vi "create_full_request_data.vi"(0 "llm_openai_chatmodels in":refnum<class "llm_gemini_chatmodels.lvclass">, 5 "Messages":refnum<class "abstract_message_base.lvclass">[](array[class]), 11 "error in (no error)":errorcluster) -> (4 "llm_openai_chatmodels out":refnum<class "llm_gemini_chatmodels.lvclass">, 6 "Request Data":string, 15 "error out":errorcluster)   [LabVIEW 2020, in "llm_gemini_chatmodels.lvclass"]
uses:
  llm_gemini_chatmodels.lvclass
  C:/Users/venkatesh.chandragir/Downloads/labview-llm-libraries-users-nigharikkha-vlm_support/src/models/abstract_llm_base/abstract_llm_base.lvclass
  abstract_message_base/abstract_message_base.lvclass
  utils/gemini_chatmodel_request_data.ctl
  message_text/message_text.lvclass
  message_image/message_image.lvclass
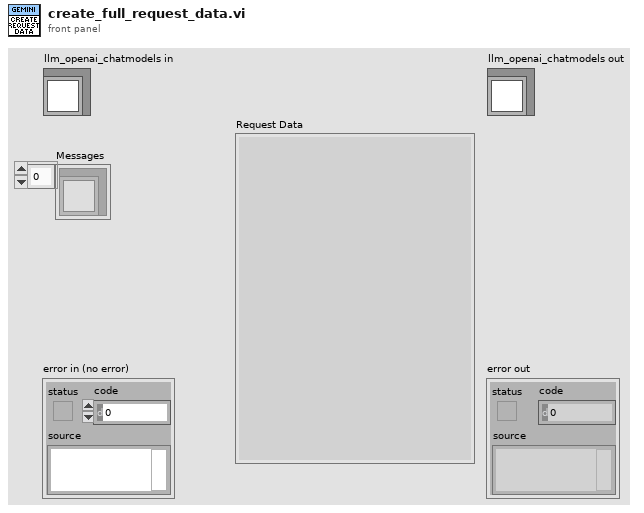
[diagram p1: front panel]
types:
  T1 = cluster{"role":string, "parts":cluster{"text":string}[]}[]
  T2 = typedef "llm_gemini_chatmodels.lvclass/gemini_chatmodel_request_data.ctl" = cluster{"contents":cluster{"role":string, "parts":cluster{"text":string}[]}[], "generation_config":cluster{"temperature":dbl, "maxOutputTokens":u32, "topP":dbl}}
  T3 = typedef "message_text.lvclass/message.ctl" = cluster{"role":string, "content":string[]}
  T4 = typedef "message_image.lvclass/message.ctl" = cluster{"role":string, "content_text":string[], "content_images":path[]}
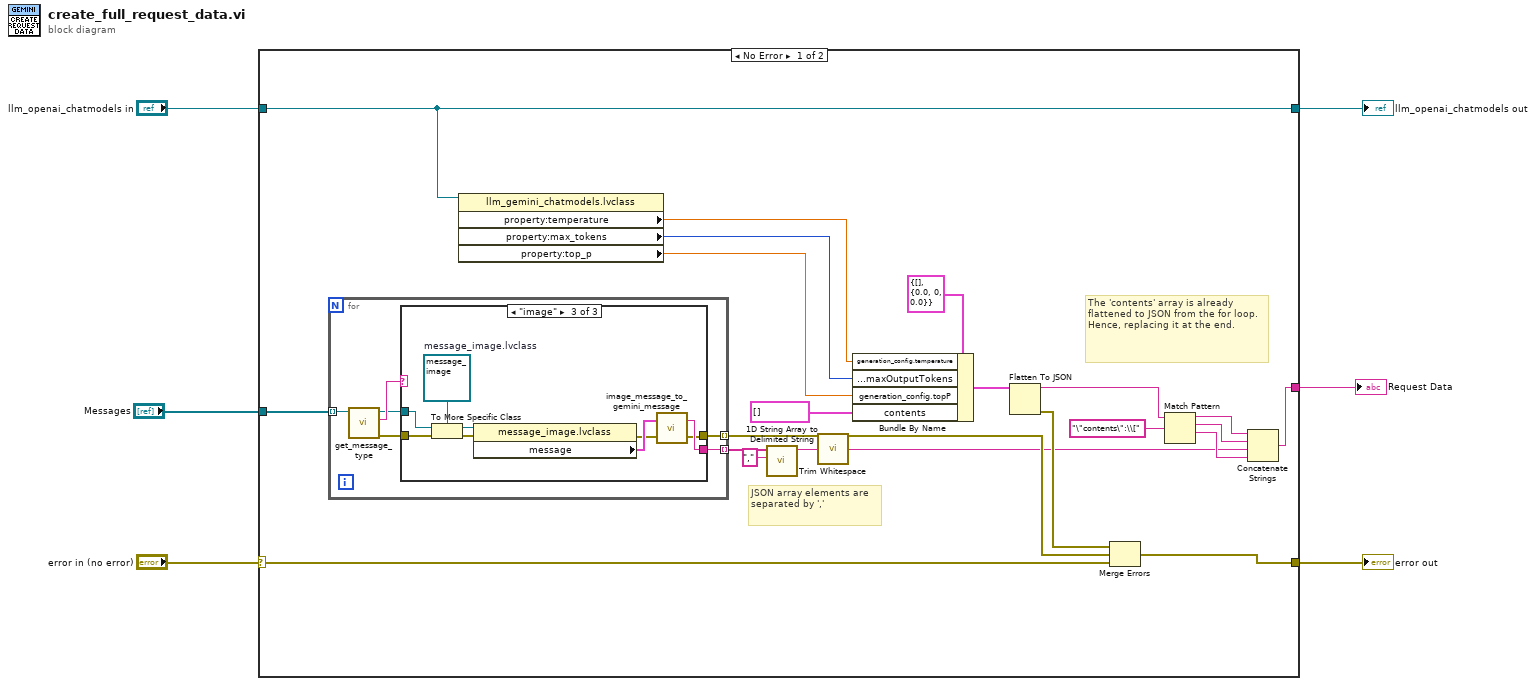
[diagram p0: block diagram]
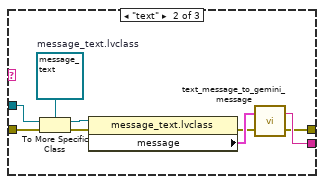
[diagram p3: hidden frame]
diagram:
  n1 = case shown="No Error" "error in (no error)" {
    selector: "error in (no error)" -> [w28 w55]
    tunnel: [w25 w55] -> w5
    tunnel: [w22 w54] -> w3
    tunnel: "llm_openai_chatmodels in" -> [w22 w54]
    tunnel: "Messages" -> [w27 _]
    tunnel: [w11 _] -> w1
    frame No Error {
      # "JSON array elements are separated by ','"
      # "The 'contents' array is already flattened to JSON from the for loop.\nHence, replacing it at the end."
      n2 = for {
        tunnel: w27 -> [w34] mode=indexing
        tunnel: [w30] -> w24 mode=indexing
        tunnel: [w29] -> w8 mode=indexing
        n3 = call-dynamic "get_message_type.vi"("abstract_message_base in"=w34) -> ("error out"=w31:errorcluster, "Type"=w33:string, "abstract_message_base out"=w32:refnum<class "abstract_message_base.lvclass">)  [unwired: 8 in]
        n4 = case shown="\"image\"" w33 {
          tunnel: w32 -> [_ w43 w52]
          tunnel: w31 -> [w35 w44 w53]
          tunnel: [w35 w36 w45] -> w30
          tunnel: [_ w38 w47] -> w29
          frame Default {
          }
          frame "text" {
            w42 = refnum<class "message_text.lvclass"> refnum  # message_text.lvclass
            n5 = To More Specific Class(target class=w42, reference=w43, error in=w44) -> (specific class reference=w41:refnum<class "message_text.lvclass">, error out=w40:errorcluster)
            n6 = property class="message_text.lvclass"(reference=w41, error in=w40) -> (error out=w37:errorcluster, "message"=w39:T3)  [unwired: 1 out]
            n7 = call "text_message_to_gemini_message.vi"("error in (no error)"=w37, "message"=w39) -> ("error out"=w36:errorcluster, "Content (JSON)"=w38:string)
          }
          frame "image" {
            w49 = refnum<class "message_image.lvclass"> refnum  # message_image.lvclass
            n8 = To More Specific Class(target class=w49, reference=w52, error in=w53) -> (specific class reference=w51:refnum<class "message_image.lvclass">, error out=w50:errorcluster)
            n9 = property class="message_image.lvclass"(reference=w51, error in=w50) -> (error out=w46:errorcluster, "message"=w48:T4)  [unwired: 1 out]
            n10 = call "image_message_to_gemini_message.vi"("error in (no error)"=w46, "message"=w48) -> ("error out"=w45:errorcluster, "Content (JSON)"=w47:string)
          }
        }
      }
      n11 = property class="llm_gemini_chatmodels.lvclass"(reference=w22) -> ("property:temperature"=w21:dbl, "property:max_tokens"=w20:u32, "property:top_p"=w19:dbl)  [unwired: 1 in, 2 out]
      n12 = call <vilib>:"1D String Array to Delimited String.vi"("delimiter"=",", "string array"=w8) -> ("delimited string"=w9:string)  [unwired: 9 in]
      n13 = call <vilib>:"Trim Whitespace.vi"("string"=w9) -> ("trimmed string"=w7:string)  [unwired: 1 in]
      n14 = Bundle By Name(cluster=T2 {"contents"=[], "generation_config"={"temperature"=0.0, "maxOutputTokens"=0, "topP"=0.0}} ("data"), "generation_config.temperature"=w21, "generation_config.maxOutputTokens"=w20, "generation_config.topP"=w19, "contents"=T1 []) -> (w26:T2)
      n15 = Flatten To JSON(anything=w26) -> (JSON string=w12:string, 11:w23:errorcluster)  [unwired: 2 in]
      n16 = Merge Errors(w23, w24, w28) -> (w25:errorcluster)
      n17 = Match Pattern(string=w12, regular expression="\"contents\":\\[") -> (before substring=w16:string, match substring=w15:string, after substring=w14:string)  [unwired: 1 in, 1 out]
      n18 = Concatenate Strings(w16, w15, w7, w14) -> (w11:string)
    }
    frame Error {
    }
  }
  "error out" <- w5
  "llm_openai_chatmodels out" <- w3
  "Request Data" <- w1
